vi "Check Valid Message.vi"(8 "error in (no error)":errorcluster, 10 "Message":string, 11 "controller in":refnum<class "LC Parser.lvclass">) -> (0 "error out":errorcluster, 2 "Valid?":bool, 3 "controller out":refnum<class "LC Parser.lvclass">)   [LabVIEW 2020, in "LC Parser.lvclass"]
uses:
  LC Parser.lvclass
  Controller/Generic Plugin.lvclass
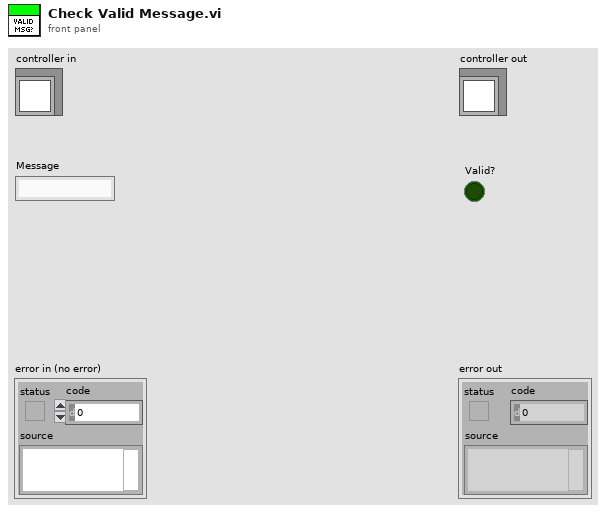
[diagram p1: front panel]
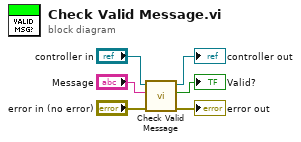
[diagram p0: block diagram]
diagram:
  n1 = call-parent "Check Valid Message.vi"("error in (no error)"="error in (no error)", "Message"="Message", "controller in"="controller in") -> ("error out"=→"error out":errorcluster, "Valid?"=→"Valid?":bool, "controller out"=→"controller out":refnum<class "LC Parser.lvclass">)  [unwired: 6 in]
